vi "CMD_07T_SetRamp.vi"(8 "Ramp speed, K/min":dbl=5.0 min=0.1 max=10.0, 9 "Target, K":dbl=295.0 min=195.0 max=400.0, 11 "VISA resource name":refnum<visa-resource-name>) -> (3 "VISA resource name out":refnum<visa-resource-name>)   [LabVIEW 2017]
panel:
  out "unsigned 16bit integer":u16
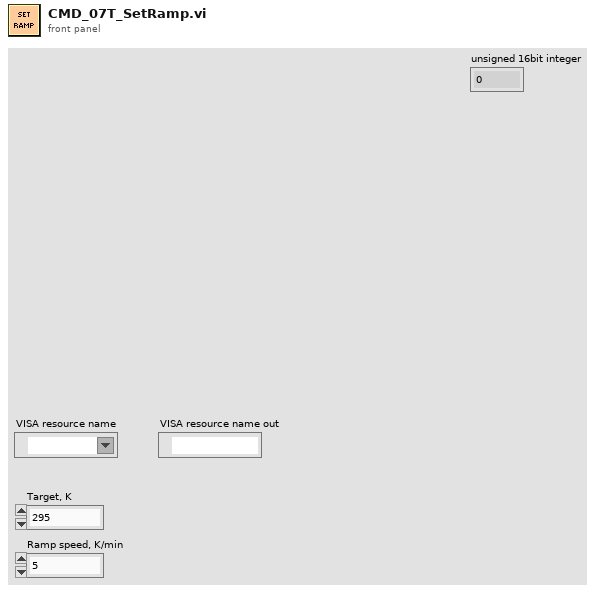
[diagram p1: front panel]
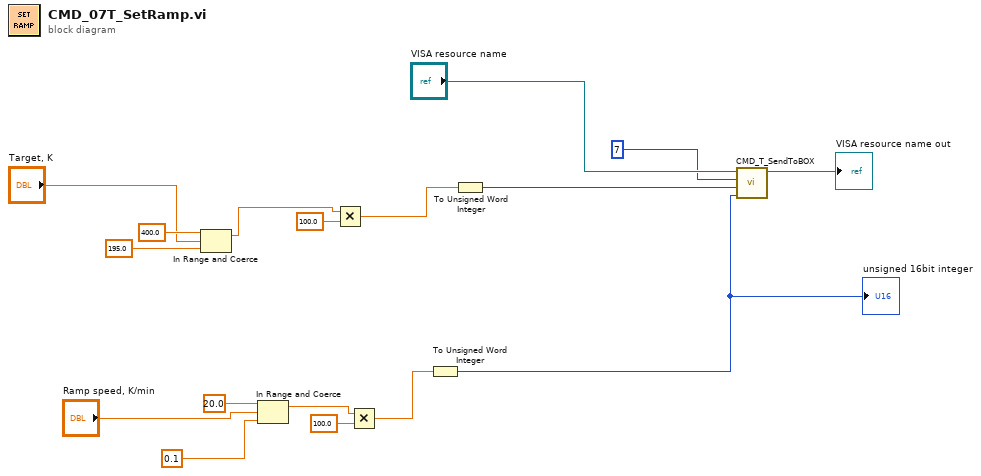
[diagram p0: block diagram]
diagram:
  n1 = In Range and Coerce(upper limit=400.0, x="Target, K", lower limit=195.0) -> (coerced(x)=w8:dbl)  [unwired: 1 out]
  n2 = In Range and Coerce(upper limit=20.0, x="Ramp speed, K/min", lower limit=0.1) -> (coerced(x)=w3:dbl)  [unwired: 1 out]
  n3 = Multiply(x=w8, y=100.0) -> (x*y=w13:dbl)
  n4 = Multiply(x=w3, y=100.0) -> (x*y=w2:dbl)
  n5 = To Unsigned Word Integer(number=w2) -> (unsigned 16bit integer=w1:u16)
  "unsigned 16bit integer" <- w1
  n6 = To Unsigned Word Integer(number=w13) -> (unsigned 16bit integer=w15:u16)
  n7 = call "CMD_T_SendToBOX.vi"("arg2"=w1, "arg1"=w15, "CMD"=i8 7, "VISA resource name"="VISA resource name") -> ("VISA resource name out"=→"VISA resource name out":refnum<visa-resource-name>)  [unwired: 7 in]
